vi "Stop AC Source.vi"(8 "error in (no error)":errorcluster, 9 "AC sync source":T1, 11 "AC source":T1) -> (0 "error out":errorcluster, 1 "AC sync source out":T1, 3 "AC source out":T1)   [LabVIEW 2020]
doc: "Stop output of the AC source and close communication."
uses:
  Type definitions/AC Source.ctl
  Type definitions/AC Source type.ctl
  <vilib>/Instr/_visa.llb/VISA GPIB Control REN Mode.ctl
  external libraries/Fluke 5XXX Series Multicalibrator/Fluke 5XXX Series Multicalibrators.lvlib
  external libraries/AWG/AFG3000/Tektronix AFG 3000 Series.lvlib
  external libraries/AWG/Agilent 33XXX Series/Agilent 33XXX Series.lvlib
panel:
  out "status":string
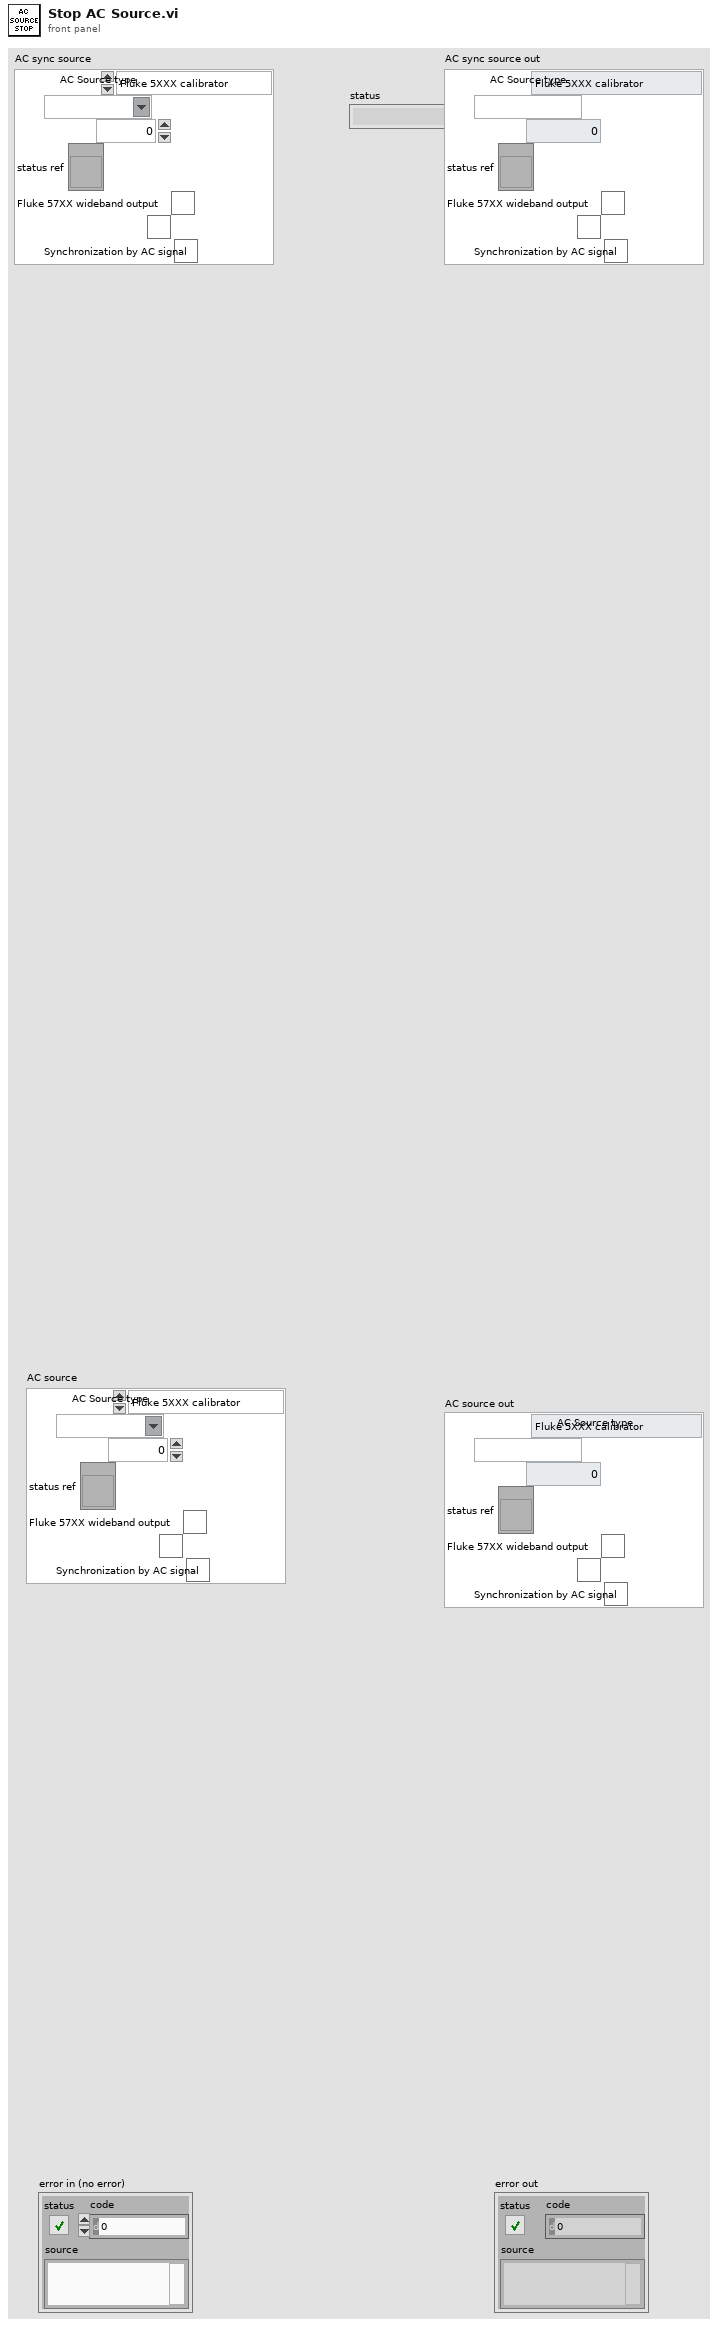
[diagram p1: front panel]
types:
  T1 = typedef "AC Source.ctl" = cluster{"AC Source type":T2, "VISA":refnum<visa-resource-name>, "Ref. clock (Hz)":dbl, "status ref":refnum<vi>, "Fluke 57XX wideband output":bool, "Fluke 57XX ignore errors":bool, "Synchronization by AC signal":bool}
  T2 = typedef "AC Source type.ctl" = enum16{"Fluke 5XXX calibrator", "Tektronix AFG3000 series", "dummy", "Agilent 331xxA to 332xxA", "Agilent 335xxA to 336xxA"}
  T3 = typedef "VISA GPIB Control REN Mode.ctl" = u16
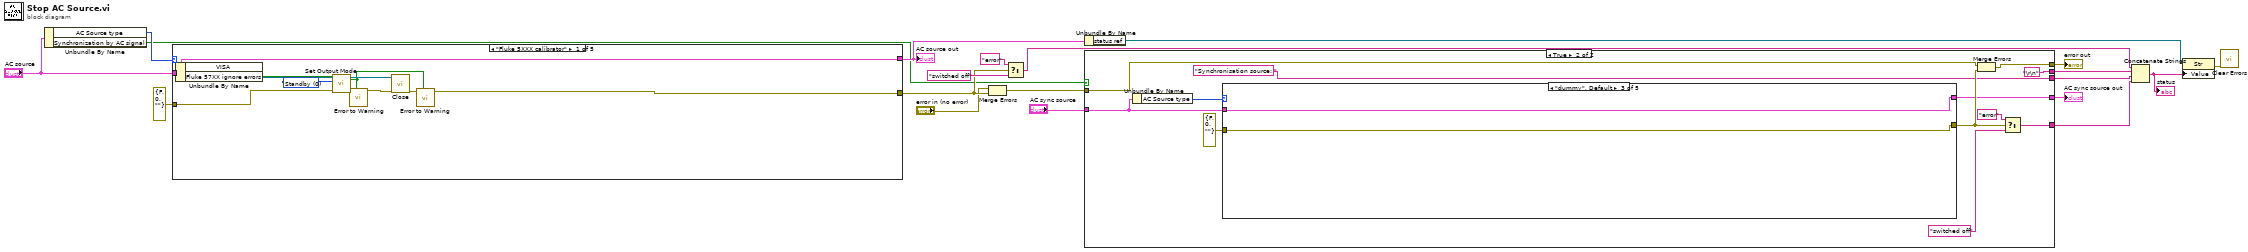
[diagram p0: block diagram]
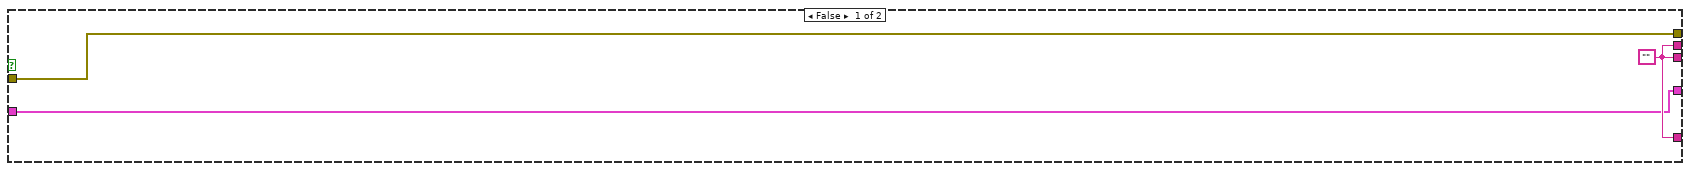
[diagram p2: hidden frame]
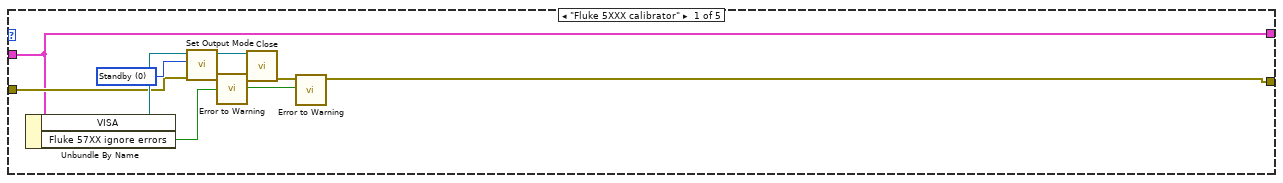
[diagram p3: hidden frame]
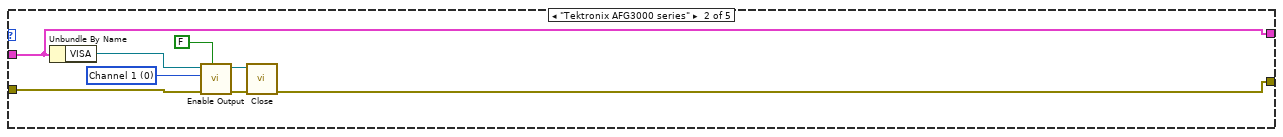
[diagram p4: hidden frame]
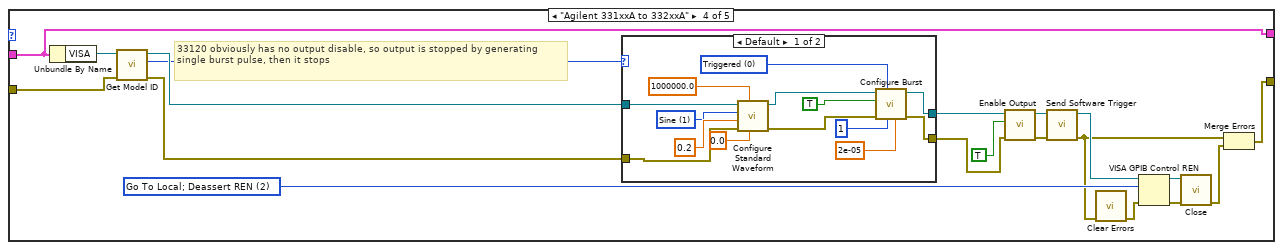
[diagram p5: hidden frame]
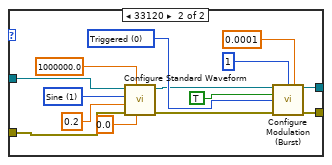
[diagram p6: hidden frame]
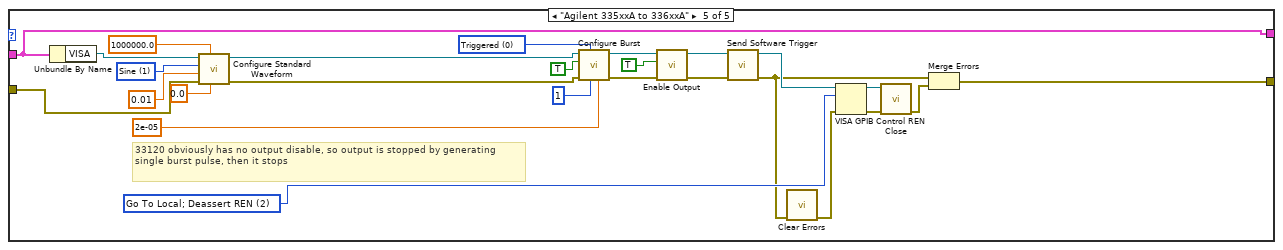
[diagram p7: hidden frame]
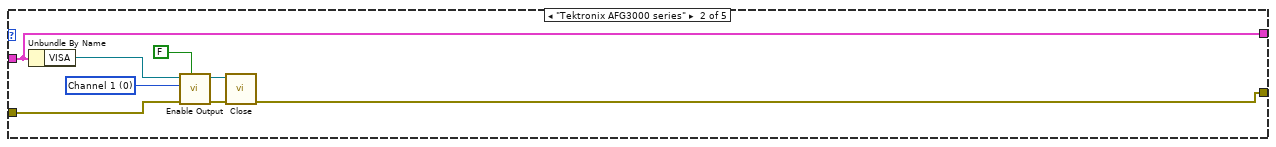
[diagram p8: hidden frame]
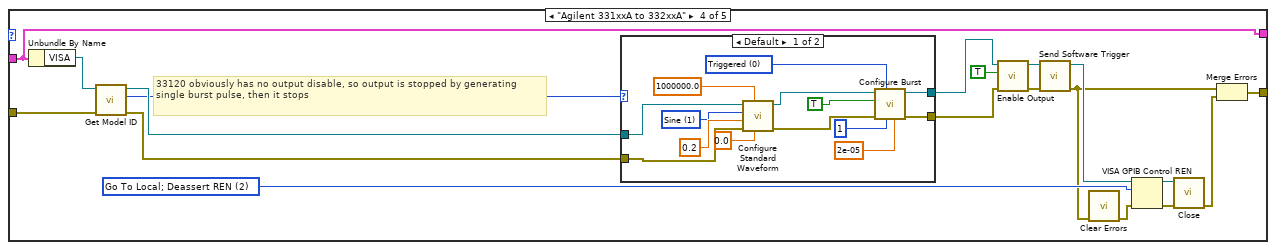
[diagram p10: hidden frame]
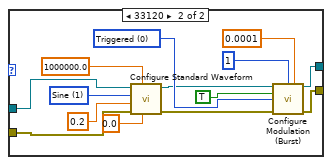
[diagram p11: hidden frame]
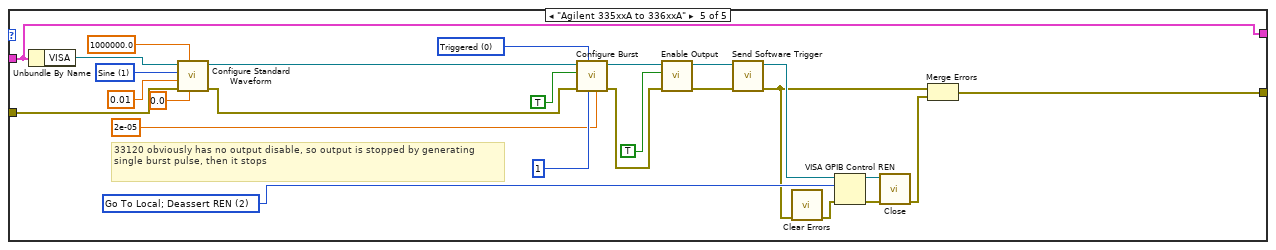
[diagram p12: hidden frame]
diagram:
  n1 = Unbundle By Name("AC source") -> ("AC Source type"=w20:T2, "Synchronization by AC signal"=w10:bool)
  n2 = case shown="\"Fluke 5XXX calibrator\"" w20 {
    tunnel: errorcluster {"status"=FALSE, "code"=0, "source"=""} ("error in (no error)") -> [w27 w37 w39 w42 w89]
    tunnel: [w24 w32 w39 w54 w108] -> w16
    tunnel: "AC source" -> [w26 w31 w40 w53 w107]
    tunnel: [w26 w31 w40 w53 w107] -> w13
    frame "Fluke 5XXX calibrator" {
      w30 = u32 0 items=["Standby", "Operate"] ("Output Mode (0: Standby)")
      n3 = Unbundle By Name(w26) -> ("VISA"=w28:refnum<visa-resource-name>, "Fluke 57XX ignore errors"=w21:bool)
      n4 = call "Set Output Mode.vi"("error in (no error)"=w27, "Output Mode (0: Standby)"=w30, "VISA resource name"=w28) -> ("error out"=w23:errorcluster, "VISA resource name out"=w29:refnum<visa-resource-name>)  [unwired: 7 in]
      n5 = call "Error to Warning.vi"("Change to warning?"=w21, "error in (no error)"=w23) -> ("error out"=w22:errorcluster)  [unwired: 9 in]
      n6 = call "Close.vi"("VISA resource name"=w29, "error in (no error)"=w22) -> ("error out"=w25:errorcluster)  [unwired: 13 in]
      n7 = call "Error to Warning.vi"("Change to warning?"=w21, "error in (no error)"=w25) -> ("error out"=w24:errorcluster)  [unwired: 9 in]
    }
    frame "Tektronix AFG3000 series" {
      w35 = u16 0 items=["Channel 1", "Channel2"] ("Channel (0: Channel 1)")
      n8 = Unbundle By Name(w31) -> ("VISA"=w36:refnum<visa-resource-name>)
      n9 = call "Enable Output.vi"("Enable Output (T: Enable)"=FALSE, "error in (no error)"=w37, "Channel (0: Channel 1)"=w35, "VISA resource name"=w36) -> ("error out"=w34:errorcluster, "VISA resource name out"=w33:refnum<visa-resource-name>)  [unwired: 6 in]
      n10 = call "Close.vi"("error in (no error)"=w34, "VISA resource name"=w33) -> ("error out"=w32:errorcluster)  [unwired: 9 in]
    }
    frame "dummy", Default {
    }
    frame "Agilent 331xxA to 332xxA" {
      w59 = T3 2 items=["Deassert REN", "Assert REN", "Go To Local; Deassert REN ", "Assert REN; Address Device", "Local Lockout (Addressed Devices)", "Local Lockout (This Device)", "Go To Local"] ("Mode")
      # "33120 obviously has no output disable, so output is stopped by generating\nsingle burst pulse, then it stops"
      n11 = Unbundle By Name(w53) -> ("VISA"=w44:refnum<visa-resource-name>)
      n12 = call "Get Model ID.vi"("error in (no error)"=w42, "VISA resource name"=w44) -> ("error out"=w52:errorcluster, "model ID"=w50:u32, "VISA resource name out"=w51:refnum<visa-resource-name>)  [unwired: 7 in]
      n13 = case shown="Default" w50 {
        tunnel: [w69 w83] -> w48
        tunnel: [w68 w82] -> w47
        tunnel: w52 -> [w63 w81]
        tunnel: w51 -> [w62 w80]
        frame Default {
          w65 = u16 1 items=["DC", "Sine", "Square", "Triangle", "Ramp", "Pulse", "Noise", "Sinc", "Negative Ramp", "Exponential Rise", "Exponential Fall", "Cardiac"] ("Waveform Function (1: Sine)")
          w73 = u16 0 items=["Triggered", "Gated"] ("Burst Mode (0: Triggered)")
          n14 = call "Configure Standard Waveform.vi"("DC Offset (0.00 V)"=0.0, "Frequency (1000 Hz)"=1000000.0, "error in (no error)"=w63, "Amplitude (1)"=0.2, "Waveform Function (1: Sine)"=w65, "VISA resource name"=w62) -> ("error out"=w61:errorcluster, "VISA resource name out"=w60:refnum<visa-resource-name>)  [unwired: 4 in]
          n15 = call "Configure Burst.vi"("Burst Period (1 s)"=2e-05, "Burst Count (1)"=1, "Burst Mode (0: Triggered)"=w73, "error in (no error)"=w61, "Enable Burst (T: Enable)"=TRUE, "VISA resource name"=w60) -> ("error out"=w69:errorcluster, "VISA resource name out"=w68:refnum<visa-resource-name>)  [unwired: 4 in]
        }
        frame 33120 {
          w76 = u16 1 items=["DC", "Sine", "Square", "Triangle", "Ramp", "Pulse", "Noise", "Sinc", "Negative Ramp", "Exponential Rise", "Exponential Fall", "Cardiac"] ("Waveform Function (1: Sine)")
          w84 = u16 0 items=["Triggered", "Gated"] ("Burst Modulation Mode (0: Triggered)")
          n16 = call "Configure Standard Waveform.vi"("DC Offset (0.00 V)"=0.0, "Frequency (1000 Hz)"=1000000.0, "error in (no error)"=w81, "Amplitude (1)"=0.2, "Waveform Function (1: Sine)"=w76, "VISA resource name"=w80) -> ("error out"=w79:errorcluster, "VISA resource name out"=w78:refnum<visa-resource-name>)  [unwired: 4 in]
          n17 = call "Configure Modulation (Burst).vi"("VISA resource name"=w78, "Burst Count (1)"=1, "Burst Period (1 s)"=0.0001, "Enable Burst Modulation (T: Enable)"=TRUE, "Burst Modulation Mode (0: Triggered)"=w84, "error in (no error)"=w79) -> ("VISA resource name out"=w82:refnum<visa-resource-name>, "error out"=w83:errorcluster)  [unwired: 8 in]
        }
      }
      n18 = call "Enable Output.vi"("error in (no error)"=w48, "Enable Output  (T: Enable)"=TRUE, "VISA resource name"=w47) -> ("error out"=w46:errorcluster, "VISA resource name out"=w45:refnum<visa-resource-name>)  [unwired: 7 in]
      n19 = call "Send Software Trigger.vi"("error in (no error)"=w46, "VISA resource name"=w45) -> ("error out"=w41:errorcluster, "VISA resource name out"=w43:refnum<visa-resource-name>)  [unwired: 8 in]
      n20 = call <vilib>:"Clear Errors.vi"("error in (no error)"=w41) -> ("error out"=w57:errorcluster)  [unwired: 5 in, 1 out]
      n21 = VISA GPIB Control REN(8:w57, 10:w59, 11:w43) -> (0:w56:errorcluster, 3:w58:refnum<visa-resource-name>)
      n22 = call "Close.vi"("error in (no error)"=w56, "VISA resource name"=w58) -> ("error out"=w55:errorcluster)  [unwired: 9 in]
      n23 = Merge Errors(w41, w55) -> (w54:errorcluster)
    }
    frame "Agilent 335xxA to 336xxA" {
      w95 = u16 1 items=["DC", "Sine", "Square", "Triangle", "Ramp", "Pulse", "Noise", "Sinc", "Negative Ramp", "Exponential Rise", "Exponential Fall", "Cardiac"] ("Waveform Function (1: Sine)")
      w101 = u16 0 items=["Triggered", "Gated"] ("Burst Mode (0: Triggered)")
      w111 = T3 2 items=["Deassert REN", "Assert REN", "Go To Local; Deassert REN ", "Assert REN; Address Device", "Local Lockout (Addressed Devices)", "Local Lockout (This Device)", "Go To Local"] ("Mode")
      # "33120 obviously has no output disable, so output is stopped by generating\nsingle burst pulse, then it stops"
      n24 = Unbundle By Name(w107) -> ("VISA"=w91:refnum<visa-resource-name>)
      n25 = call "Configure Standard Waveform.vi"("DC Offset (0.00 V)"=0.0, "Frequency (1000 Hz)"=1000000.0, "error in (no error)"=w89, "Amplitude (1)"=0.01, "Waveform Function (1: Sine)"=w95, "VISA resource name"=w91) -> ("error out"=w93:errorcluster, "VISA resource name out"=w92:refnum<visa-resource-name>)  [unwired: 4 in]
      n26 = call "Configure Burst.vi"("Burst Period (1 s)"=2e-05, "Burst Count (1)"=1, "Burst Mode (0: Triggered)"=w101, "error in (no error)"=w93, "Enable Burst (T: Enable)"=TRUE, "VISA resource name"=w92) -> ("error out"=w105:errorcluster, "VISA resource name out"=w104:refnum<visa-resource-name>)  [unwired: 4 in]
      n27 = call "Enable Output.vi"("error in (no error)"=w105, "Enable Output  (T: Enable)"=TRUE, "VISA resource name"=w104) -> ("error out"=w103:errorcluster, "VISA resource name out"=w102:refnum<visa-resource-name>)  [unwired: 7 in]
      n28 = call "Send Software Trigger.vi"("error in (no error)"=w103, "VISA resource name"=w102) -> ("error out"=w88:errorcluster, "VISA resource name out"=w90:refnum<visa-resource-name>)  [unwired: 8 in]
      n29 = call <vilib>:"Clear Errors.vi"("error in (no error)"=w88) -> ("error out"=w110:errorcluster)  [unwired: 5 in, 1 out]
      n30 = VISA GPIB Control REN(8:w110, 10:w111, 11:w90) -> (0:w113:errorcluster, 3:w112:refnum<visa-resource-name>)
      n31 = call "Close.vi"("error in (no error)"=w113, "VISA resource name"=w112) -> ("error out"=w109:errorcluster)  [unwired: 9 in]
      n32 = Merge Errors(w88, w109) -> (w108:errorcluster)
    }
  }
  "AC source out" <- w13
  n33 = Merge Errors("error in (no error)", w16) -> (w8:errorcluster)
  n34 = Select(t="error" ("idn string"), s=w16, f="switched off" ("idn string")) -> (s? t:f=w5:string)
  n35 = Unbundle By Name(w13) -> ("status ref"=w12:refnum<vi>)
  n36 = case shown="True" w10 {
    tunnel: "AC sync source" -> [w114 w126]
    tunnel: w8 -> [w115 w123]
    tunnel: [w114 w121] -> w7
    tunnel: [w115 w120] -> w6
    tunnel: [w116 "Synchronisation source: " ("string")] -> w3
    tunnel: [w116 "\r\n"] -> w2
    tunnel: [w116 w117] -> w1
    frame False {
      w116 = ""
    }
    frame True {
      n37 = Unbundle By Name(w126) -> ("AC Source type"=w127:T2)
      n38 = case shown="\"dummy\", Default" w127 {
        tunnel: errorcluster {"status"=FALSE, "code"=0, "source"=""} ("error in (no error)") -> [w135 w145 w147 w150 w197]
        tunnel: [w130 w140 w147 w162 w216] -> w122
        tunnel: w126 -> [w134 w139 w148 w161 w215]
        tunnel: [w134 w139 w148 w161 w215] -> w121
        frame "Fluke 5XXX calibrator" {
          w138 = u32 0 items=["Standby", "Operate"] ("Output Mode (0: Standby)")
          n39 = Unbundle By Name(w134) -> ("VISA"=w136:refnum<visa-resource-name>, "Fluke 57XX ignore errors"=w129:bool)
          n40 = call "Set Output Mode.vi"("error in (no error)"=w135, "Output Mode (0: Standby)"=w138, "VISA resource name"=w136) -> ("error out"=w133:errorcluster, "VISA resource name out"=w137:refnum<visa-resource-name>)  [unwired: 7 in]
          n41 = call "Error to Warning.vi"("Change to warning?"=w129, "error in (no error)"=w133) -> ("error out"=w132:errorcluster)  [unwired: 9 in]
          n42 = call "Close.vi"("VISA resource name"=w137, "error in (no error)"=w132) -> ("error out"=w131:errorcluster)  [unwired: 13 in]
          n43 = call "Error to Warning.vi"("Change to warning?"=w129, "error in (no error)"=w131) -> ("error out"=w130:errorcluster)  [unwired: 9 in]
        }
        frame "Tektronix AFG3000 series" {
          w143 = u16 0 items=["Channel 1", "Channel2"] ("Channel (0: Channel 1)")
          n44 = Unbundle By Name(w139) -> ("VISA"=w144:refnum<visa-resource-name>)
          n45 = call "Enable Output.vi"("Enable Output (T: Enable)"=FALSE, "error in (no error)"=w145, "Channel (0: Channel 1)"=w143, "VISA resource name"=w144) -> ("error out"=w142:errorcluster, "VISA resource name out"=w141:refnum<visa-resource-name>)  [unwired: 6 in]
          n46 = call "Close.vi"("error in (no error)"=w142, "VISA resource name"=w141) -> ("error out"=w140:errorcluster)  [unwired: 9 in]
        }
        frame "dummy", Default {
        }
        frame "Agilent 331xxA to 332xxA" {
          w167 = T3 2 items=["Deassert REN", "Assert REN", "Go To Local; Deassert REN ", "Assert REN; Address Device", "Local Lockout (Addressed Devices)", "Local Lockout (This Device)", "Go To Local"] ("Mode")
          # "33120 obviously has no output disable, so output is stopped by generating\nsingle burst pulse, then it stops"
          n47 = Unbundle By Name(w161) -> ("VISA"=w152:refnum<visa-resource-name>)
          n48 = call "Get Model ID.vi"("error in (no error)"=w150, "VISA resource name"=w152) -> ("error out"=w160:errorcluster, "model ID"=w158:u32, "VISA resource name out"=w159:refnum<visa-resource-name>)  [unwired: 7 in]
          n49 = case shown="Default" w158 {
            tunnel: [w177 w191] -> w156
            tunnel: [w176 w190] -> w155
            tunnel: w160 -> [w171 w189]
            tunnel: w159 -> [w170 w188]
            frame Default {
              w173 = u16 1 items=["DC", "Sine", "Square", "Triangle", "Ramp", "Pulse", "Noise", "Sinc", "Negative Ramp", "Exponential Rise", "Exponential Fall", "Cardiac"] ("Waveform Function (1: Sine)")
              w181 = u16 0 items=["Triggered", "Gated"] ("Burst Mode (0: Triggered)")
              n50 = call "Configure Standard Waveform.vi"("DC Offset (0.00 V)"=0.0, "Frequency (1000 Hz)"=1000000.0, "error in (no error)"=w171, "Amplitude (1)"=0.2, "Waveform Function (1: Sine)"=w173, "VISA resource name"=w170) -> ("error out"=w169:errorcluster, "VISA resource name out"=w168:refnum<visa-resource-name>)  [unwired: 4 in]
              n51 = call "Configure Burst.vi"("Burst Period (1 s)"=2e-05, "Burst Count (1)"=1, "Burst Mode (0: Triggered)"=w181, "error in (no error)"=w169, "Enable Burst (T: Enable)"=TRUE, "VISA resource name"=w168) -> ("error out"=w177:errorcluster, "VISA resource name out"=w176:refnum<visa-resource-name>)  [unwired: 4 in]
            }
            frame 33120 {
              w184 = u16 1 items=["DC", "Sine", "Square", "Triangle", "Ramp", "Pulse", "Noise", "Sinc", "Negative Ramp", "Exponential Rise", "Exponential Fall", "Cardiac"] ("Waveform Function (1: Sine)")
              w192 = u16 0 items=["Triggered", "Gated"] ("Burst Modulation Mode (0: Triggered)")
              n52 = call "Configure Standard Waveform.vi"("DC Offset (0.00 V)"=0.0, "Frequency (1000 Hz)"=1000000.0, "error in (no error)"=w189, "Amplitude (1)"=0.2, "Waveform Function (1: Sine)"=w184, "VISA resource name"=w188) -> ("error out"=w187:errorcluster, "VISA resource name out"=w186:refnum<visa-resource-name>)  [unwired: 4 in]
              n53 = call "Configure Modulation (Burst).vi"("VISA resource name"=w186, "Burst Count (1)"=1, "Burst Period (1 s)"=0.0001, "Enable Burst Modulation (T: Enable)"=TRUE, "Burst Modulation Mode (0: Triggered)"=w192, "error in (no error)"=w187) -> ("VISA resource name out"=w190:refnum<visa-resource-name>, "error out"=w191:errorcluster)  [unwired: 8 in]
            }
          }
          n54 = call "Enable Output.vi"("error in (no error)"=w156, "Enable Output  (T: Enable)"=TRUE, "VISA resource name"=w155) -> ("error out"=w154:errorcluster, "VISA resource name out"=w153:refnum<visa-resource-name>)  [unwired: 7 in]
          n55 = call "Send Software Trigger.vi"("error in (no error)"=w154, "VISA resource name"=w153) -> ("error out"=w149:errorcluster, "VISA resource name out"=w151:refnum<visa-resource-name>)  [unwired: 8 in]
          n56 = call <vilib>:"Clear Errors.vi"("error in (no error)"=w149) -> ("error out"=w165:errorcluster)  [unwired: 5 in, 1 out]
          n57 = VISA GPIB Control REN(8:w165, 10:w167, 11:w151) -> (0:w164:errorcluster, 3:w166:refnum<visa-resource-name>)
          n58 = call "Close.vi"("error in (no error)"=w164, "VISA resource name"=w166) -> ("error out"=w163:errorcluster)  [unwired: 9 in]
          n59 = Merge Errors(w149, w163) -> (w162:errorcluster)
        }
        frame "Agilent 335xxA to 336xxA" {
          w203 = u16 1 items=["DC", "Sine", "Square", "Triangle", "Ramp", "Pulse", "Noise", "Sinc", "Negative Ramp", "Exponential Rise", "Exponential Fall", "Cardiac"] ("Waveform Function (1: Sine)")
          w209 = u16 0 items=["Triggered", "Gated"] ("Burst Mode (0: Triggered)")
          w219 = T3 2 items=["Deassert REN", "Assert REN", "Go To Local; Deassert REN ", "Assert REN; Address Device", "Local Lockout (Addressed Devices)", "Local Lockout (This Device)", "Go To Local"] ("Mode")
          # "33120 obviously has no output disable, so output is stopped by generating\nsingle burst pulse, then it stops"
          n60 = Unbundle By Name(w215) -> ("VISA"=w199:refnum<visa-resource-name>)
          n61 = call "Configure Standard Waveform.vi"("DC Offset (0.00 V)"=0.0, "Frequency (1000 Hz)"=1000000.0, "error in (no error)"=w197, "Amplitude (1)"=0.01, "Waveform Function (1: Sine)"=w203, "VISA resource name"=w199) -> ("error out"=w201:errorcluster, "VISA resource name out"=w200:refnum<visa-resource-name>)  [unwired: 4 in]
          n62 = call "Configure Burst.vi"("Burst Period (1 s)"=2e-05, "Burst Count (1)"=1, "Burst Mode (0: Triggered)"=w209, "error in (no error)"=w201, "Enable Burst (T: Enable)"=TRUE, "VISA resource name"=w200) -> ("error out"=w213:errorcluster, "VISA resource name out"=w212:refnum<visa-resource-name>)  [unwired: 4 in]
          n63 = call "Enable Output.vi"("error in (no error)"=w213, "Enable Output  (T: Enable)"=TRUE, "VISA resource name"=w212) -> ("error out"=w211:errorcluster, "VISA resource name out"=w210:refnum<visa-resource-name>)  [unwired: 7 in]
          n64 = call "Send Software Trigger.vi"("error in (no error)"=w211, "VISA resource name"=w210) -> ("error out"=w196:errorcluster, "VISA resource name out"=w198:refnum<visa-resource-name>)  [unwired: 8 in]
          n65 = call <vilib>:"Clear Errors.vi"("error in (no error)"=w196) -> ("error out"=w218:errorcluster)  [unwired: 5 in, 1 out]
          n66 = VISA GPIB Control REN(8:w218, 10:w219, 11:w198) -> (0:w221:errorcluster, 3:w220:refnum<visa-resource-name>)
          n67 = call "Close.vi"("error in (no error)"=w221, "VISA resource name"=w220) -> ("error out"=w217:errorcluster)  [unwired: 9 in]
          n68 = Merge Errors(w196, w217) -> (w216:errorcluster)
        }
      }
      n69 = Merge Errors(w123, w122) -> (w120:errorcluster)
      n70 = Select(t="error" ("idn string"), s=w122, f="switched off" ("idn string")) -> (s? t:f=w117:string)
    }
  }
  "error out" <- w6
  "AC sync source out" <- w7
  n71 = Concatenate Strings(w5, w2, w3, w1) -> (w4:string)
  "status" <- w4
  n72 = property class="Str"(reference=w12, "Value"=w4) -> (error out=w11:errorcluster)  [unwired: 1 in, 1 out]
  n73 = call <vilib>:"Clear Errors.vi"("error in (no error)"=w11) -> ()  [unwired: 5 in, 2 out]
